vi "Facade_Gauge_PUMP.vi"(0 "Data In":T6, 2 "Display State In":T4, 3 "Container State":T5) -> (6 "Data Out":T6, 7 "Display State Out":T4, 8 "Action":T3)   [LabVIEW 2019, in "Gauge_pump.xctl"]
uses:
  Gauge_pump.xctl
  Data Gauge_pump.ctl
  <vilib>/_xctls/Container State.ctl
  State _Gauge_pump.ctl
  <vilib>/_xctls/Action.ctl
  Gauge_SD.ctl
  LeftRightBoolean.ctl
  <vilib>/_xctls/XControlSupport.lvlib
panel:
  out "rotation":T1
  in  "Gauge":T2 scale=0.0..100.0
  in  "start/stop":bool
  in  "direction":bool
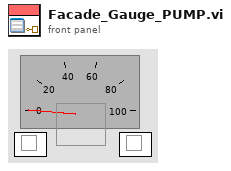
[diagram p1: front panel]
types:
  T1 = typedef "LeftRightBoolean.ctl" = bool
  T2 = typedef "Gauge_SD.ctl" = dbl
  T3 = typedef "XControlSupport.lvlib/Action.ctl" = cluster{"Data Changed?":bool, "State Changed?":bool, "Action Name":string}
  T4 = typedef "Gauge_pump.xctl/State _Gauge_pump.ctl" = cluster{"RPM":dbl, "direction":bool, "start/stop":bool, "RPMEvent":refnum<user-event>, "DirectionEvent":refnum<user-event>, "Start_stopEvent":refnum<user-event>}
  T5 = typedef "XControlSupport.lvlib/Container State.ctl" = cluster{"Indicator?":bool, "Run Mode?":bool, " Refnum":refnum<vi>}
  T6 = typedef "Gauge_pump.xctl/Data Gauge_pump.ctl" = cluster{"Data":dbl, "direction":bool, "start/stop":bool}
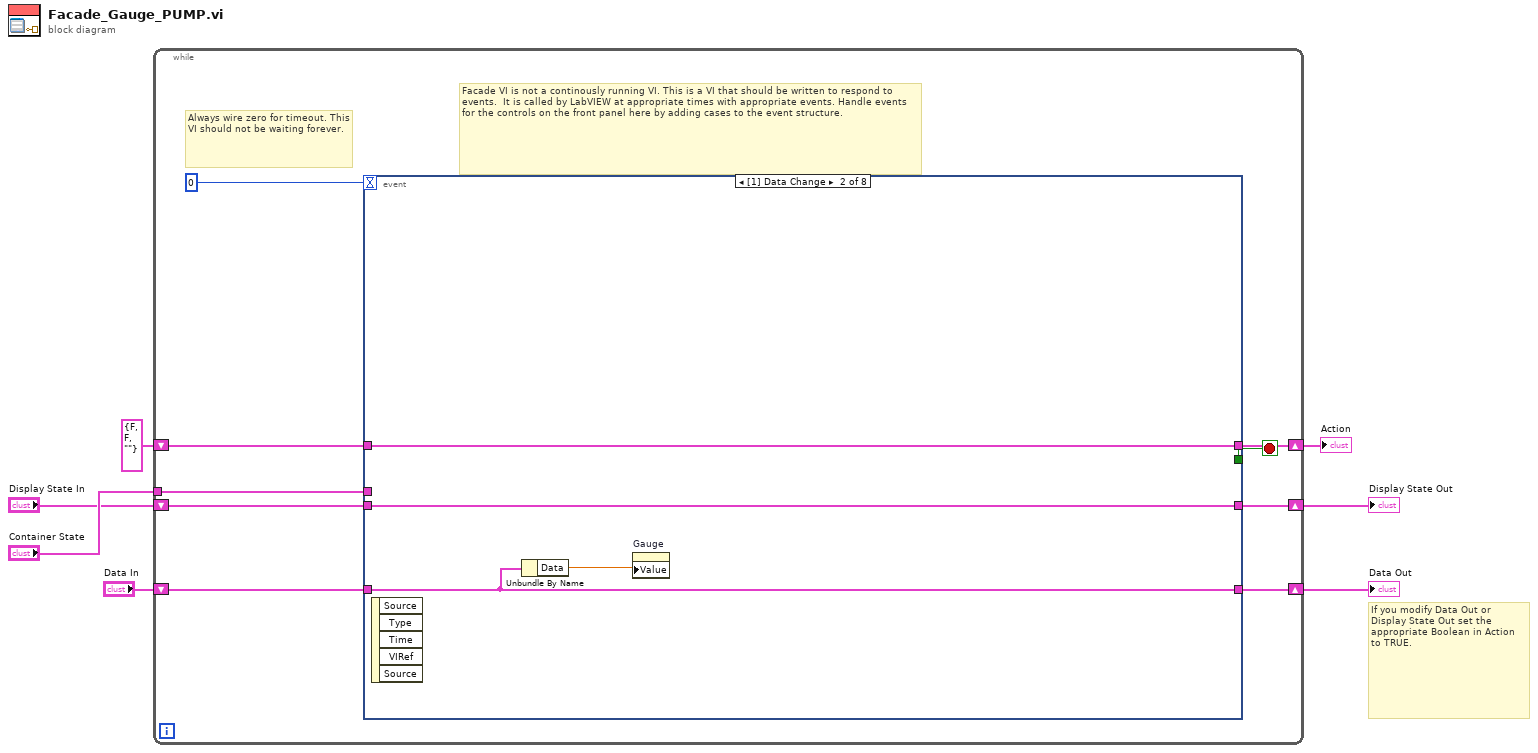
[diagram p0: block diagram]
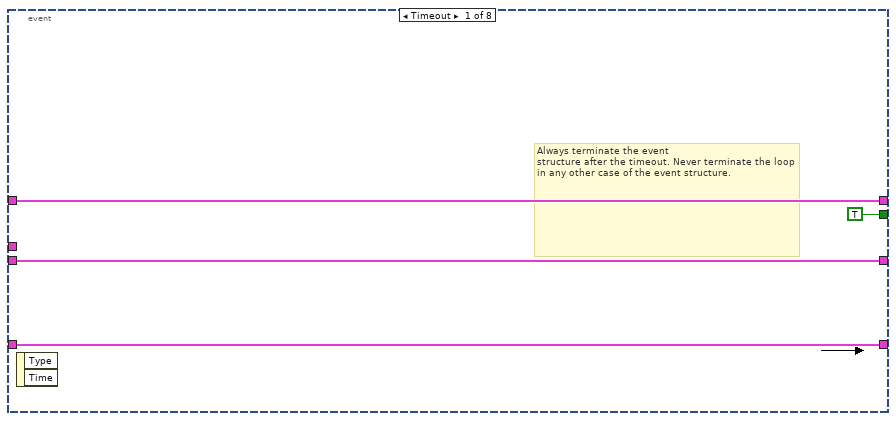
[diagram p2: hidden frame]
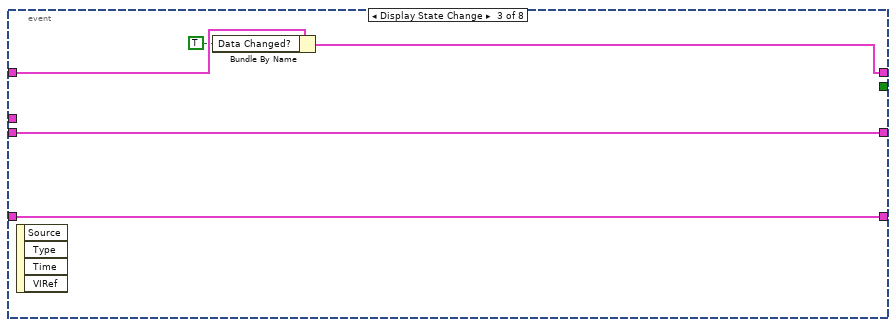
[diagram p3: hidden frame]
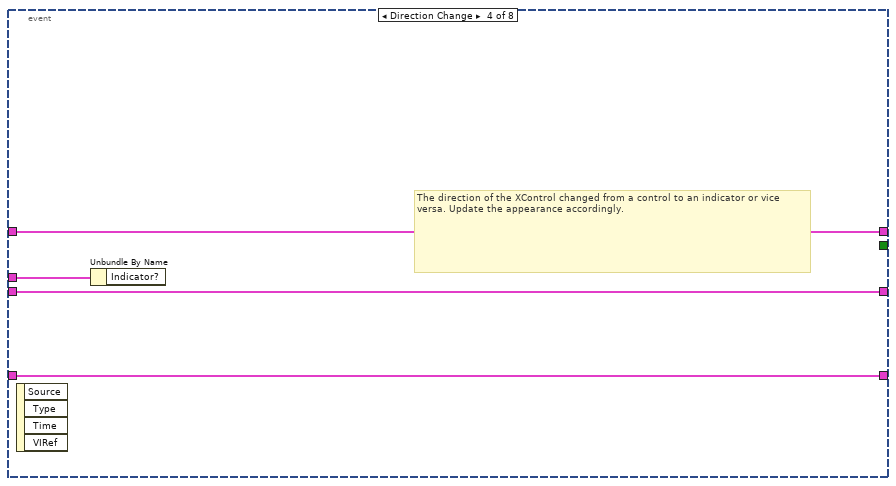
[diagram p4: hidden frame]
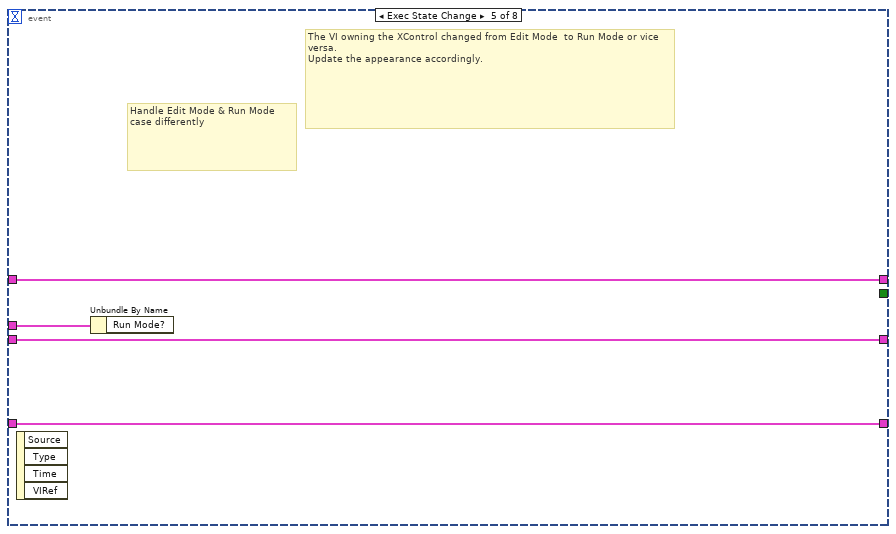
[diagram p5: hidden frame]
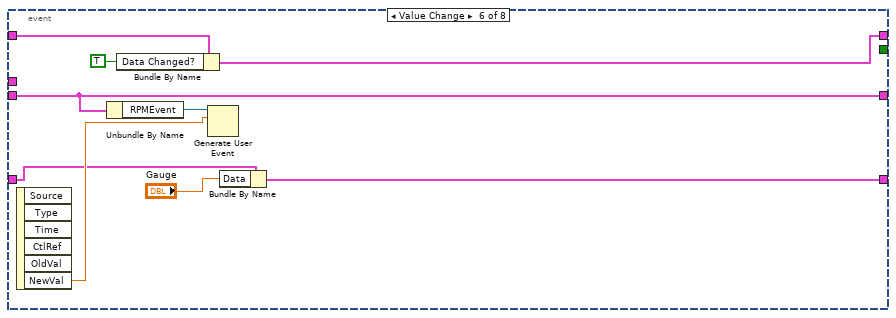
[diagram p6: hidden frame]
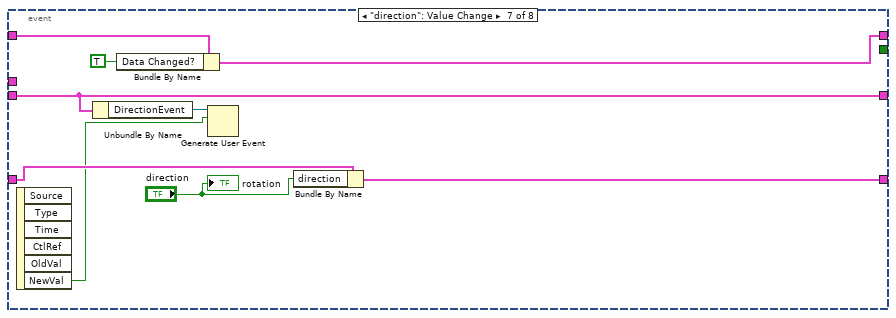
[diagram p7: hidden frame]
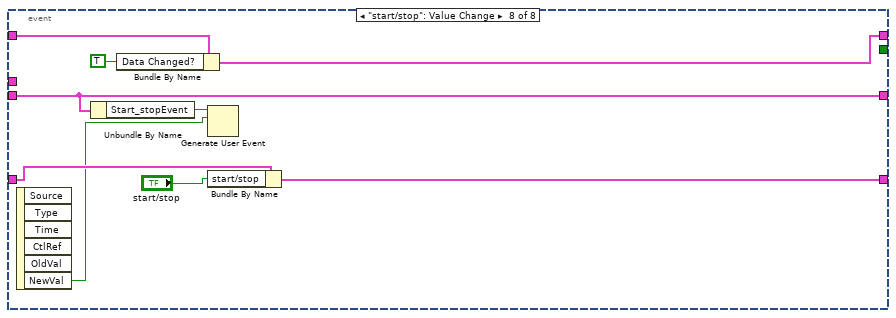
[diagram p8: hidden frame]
diagram:
  # "If you modify Data Out or\nDisplay State Out set the\nappropriate Boolean in Action\nto TRUE."
  n1 = while {
    shift-right: [w15] -> w4
    shift-left: "Display State In" -> [w16]
    tunnel: "Container State" -> [w12]
    shift-right: [w10] -> w7
    shift-left: "Data In" -> [w11]
    shift-right: [w8] -> w2
    shift-left: T3 {"Data Changed?"=FALSE, "State Changed?"=FALSE, "Action Name"=""} ("Action") -> [w9]
    stop <- w14 stop-if-true
    # "Facade VI is not a continously running VI. This is a VI that should be written to respond to events.  It is called by LabVIEW at appropriate times with appropriate events. Handle events for the controls on the front panel here by adding cases to the event structure."
    # "Always wire zero for timeout. This\nVI should not be waiting forever."
    n2 = event shown="[1] Data Change" {
      selector: _ -> [_ _ _ _ _ _ _ _]
      dyn-events: _ -> [_ _ _ _ _ _ _ _]
      timeout: 0 -> [_ _ _ _ _ _ _ _]
      tunnel: w16 -> [w18 w24 w28 w32 w36 w39 w47 w58]
      tunnel: [w18 w24 w28 w32 w36 w39 w47 w58] -> w15
      tunnel: [TRUE _ _ _ _ _ _ _] -> w14
      tunnel: w12 -> [_ _ _ w33 w37 _ _ _]
      tunnel: w11 -> [w17 w22 w29 w31 w35 w38 w52 w61]
      tunnel: [w17 w22 w29 w31 w35 w43 w51 w60] -> w10
      tunnel: [w19 w23 w25 w30 w34 w44 w53 w62] -> w8
      tunnel: w9 -> [w19 w23 w27 w30 w34 w46 w55 w64]
      event Timeout {
        # "Always terminate the event\nstructure after the timeout. Never terminate the loop in any other case of the event structure."
        n3 = event-data() -> ()  [unwired: 1 in, 2 out]
      }
      event Data Change {
        n4 = event-data() -> ()  [unwired: 1 in, 5 out]
        n5 = Unbundle By Name(w22) -> ("Data"=w21:dbl)
        n6 = property on="Gauge" class="Knob (strict)"("Value"=w21) -> ()  [unwired: 2 in, 2 out]
      }
      event Display State Change {
        n7 = event-data() -> ()  [unwired: 1 in, 4 out]
        n8 = Bundle By Name(cluster=w27, "Data Changed?"=TRUE) -> (w25:T3)
      }
      event Direction Change {
        # "The direction of the XControl changed from a control to an indicator or vice versa. Update the appearance accordingly."
        n9 = event-data() -> ()  [unwired: 1 in, 4 out]
        n10 = Unbundle By Name(w33) -> ()  [unwired: 1 out]
      }
      event Exec State Change {
        # "The VI owning the XControl changed from Edit Mode  to Run Mode or vice versa.\nUpdate the appearance accordingly."
        # "Handle Edit Mode & Run Mode\ncase differently"
        n11 = event-data() -> ()  [unwired: 1 in, 4 out]
        n12 = Unbundle By Name(w37) -> ()  [unwired: 1 out]
      }
      event Value Change {
        n13 = event-data() -> ("NewVal"=w40:T2)  [unwired: 1 in, 5 out]
        n14 = Unbundle By Name(w39) -> ("RPMEvent"=w41:refnum<user-event>)
        n15 = Bundle By Name(cluster=w46, "Data Changed?"=TRUE) -> (w44:T3)
        n16 = Generate User Event(user event=w41, event data cluster=w40) -> ()  [unwired: 2 in, 2 out]
        n17 = Bundle By Name(cluster=w38, "Data"="Gauge") -> (w43:T6)
      }
      event "direction": Value Change {
        n18 = event-data() -> ("NewVal"=w48:bool)  [unwired: 1 in, 5 out]
        n19 = Unbundle By Name(w47) -> ("DirectionEvent"=w49:refnum<user-event>)
        n20 = Bundle By Name(cluster=w55, "Data Changed?"=TRUE) -> (w53:T3)
        n21 = Generate User Event(user event=w49, event data cluster=w48) -> ()  [unwired: 2 in, 2 out]
        n22 = Bundle By Name(cluster=w52, "direction"="direction") -> (w51:T6)
        "rotation" <- "direction"
      }
      event "start/stop": Value Change {
        n23 = event-data() -> ("NewVal"=w56:bool)  [unwired: 1 in, 5 out]
        n24 = Unbundle By Name(w58) -> ("Start_stopEvent"=w57:refnum<user-event>)
        n25 = Bundle By Name(cluster=w64, "Data Changed?"=TRUE) -> (w62:T3)
        n26 = Generate User Event(user event=w57, event data cluster=w56) -> ()  [unwired: 2 in, 2 out]
        n27 = Bundle By Name(cluster=w61, "start/stop"="start/stop") -> (w60:T6)
      }
    }
  }
  "Display State Out" <- w4
  "Data Out" <- w7
  "Action" <- w2
